vi "TreeBot.vi"(8 "error in (no error)":errorcluster, 10 "Gameboard":T1, 11 "Map":T2) -> (0 "error out":errorcluster, 3 "Move":i8)   [LabVIEW 2020]
uses:
  controls/DecisionTree.ctl
  controls/Gameboard Data.ctl
  controls/DecisionTreeRecord.ctl
  controls/Player.ctl
  <vilib>/numeric/Random Number (Range).vi
  <vilib>/numeric/Random Number (Range) I64.vi
  <vilib>/numeric/sub_Random U32.vi
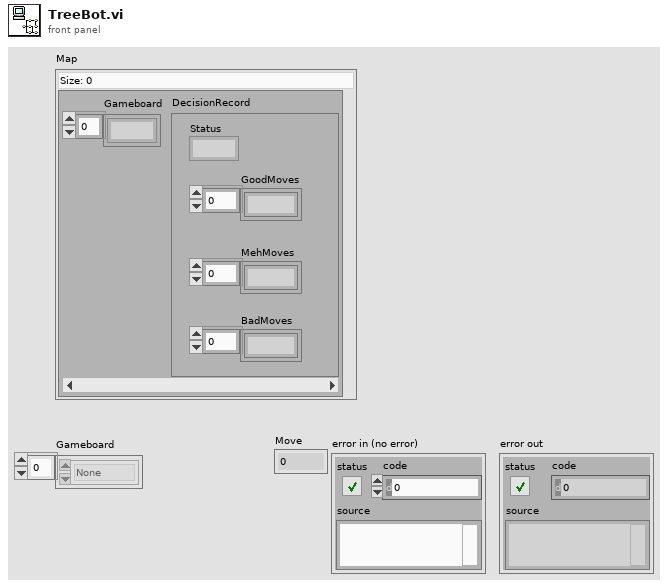
[diagram p1: front panel]
types:
  T1 = typedef "Gameboard Data.ctl" = enum16{"None", "Player 1", "Player 2"}[]
  T2 = typedef "DecisionTree.ctl" = map{T1, T3}
  T3 = typedef "DecisionTreeRecord.ctl" = cluster{"Status":T4, "GoodMoves":i8[], "MehMoves":i8[], "BadMoves":i8[]}
  T4 = typedef "Player.ctl" = enum16{"None", "Player 1", "Player 2"}
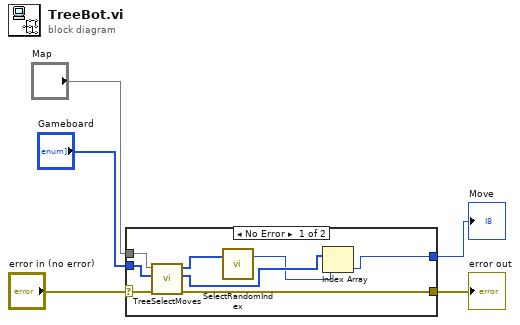
[diagram p0: block diagram]
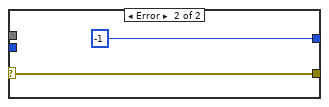
[diagram p2: hidden frame]
diagram:
  n1 = case shown="No Error" "error in (no error)" {
    selector: "error in (no error)" -> [w11 w15]
    tunnel: [w9 w15] -> w4
    tunnel: "Map" -> [w13 _]
    tunnel: "Gameboard" -> [w12 _]
    tunnel: [w6 i8 -1 ("Selected Index")] -> w1
    frame No Error {
      n2 = call "TreeSelectMoves.vi"("error in (no error)"=w11, "Gameboard"=w12, "Map"=w13) -> ("error out"=w9:errorcluster, "How rotated?"=w8:i8[], "Moves"=w10:i8[])  [unwired: 6 in]
      n3 = call "SelectRandomIndex.vi"("Indices"=w10) -> ("Selected Index"=w7:i8)  [unwired: 2 in]
      n4 = Index Array(array=w8, index=w7) -> (element=w6:i8)
    }
    frame Error {
    }
  }
  "error out" <- w4
  "Move" <- w1
